vi "Select Device List.vi"(8 "error in (no error)":errorcluster, 11 "Configuration in":refnum<class "Configuration.lvclass">) -> (0 "error out":errorcluster, 3 "Configuration out":refnum<class "Configuration.lvclass">)   [LabVIEW 2023, in "Configuration.lvlib" / "Configuration.lvclass"]
doc: "After loading the table boundaries with <b>Find Table Boundaries</b>, this routine selects the table defined by the boundaries, and stores the table in provate data for reference."
uses:
  Library/Configuration.lvclass
  Library/Configuration.lvclass/Configuration.ctl
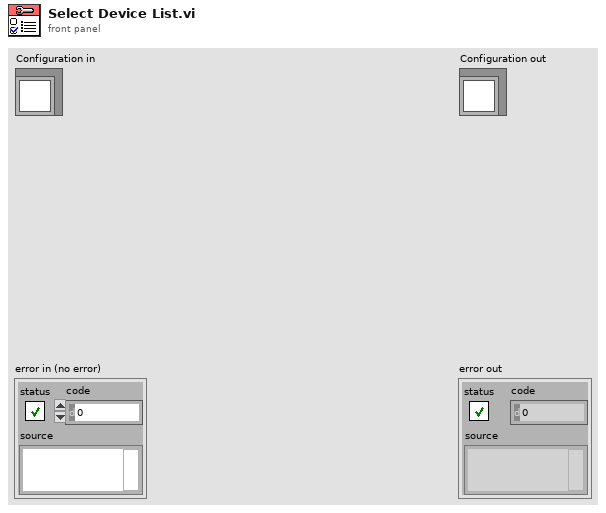
[diagram p1: front panel]
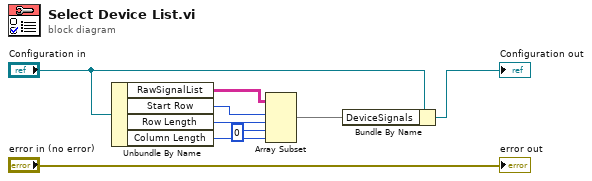
[diagram p0: block diagram]
diagram:
  n1 = Unbundle By Name("Configuration in") -> ("RawSignalList"=w8:string[][], "Start Row"=w7:i32, "Row Length"=w6:i32, "Column Length"=w5:i32)
  n2 = Array Subset(array=w8, index (row)=w7, length (row)=w6, index (col)=0 ("index"), length (col)=w5) -> (w3:string[][])
  n3 = Bundle By Name(cluster="Configuration in", "DeviceSignals"=w3) -> (→"Configuration out":refnum<class "Configuration.lvclass">)
  "error out" <- "error in (no error)"
